vi "About Robot.vi"(8 "error in (no error)":errorcluster) -> (0 "error out":errorcluster)   [LabVIEW 2011]
panel:
  in  "stop?":bool
  in  "Tab Control":T1(tab)
  # "Autonomous Mapping Robot Platform"
  # "Robot Discription Goes Here:"
  # "Laser Range \nFinder (LIDAR)"
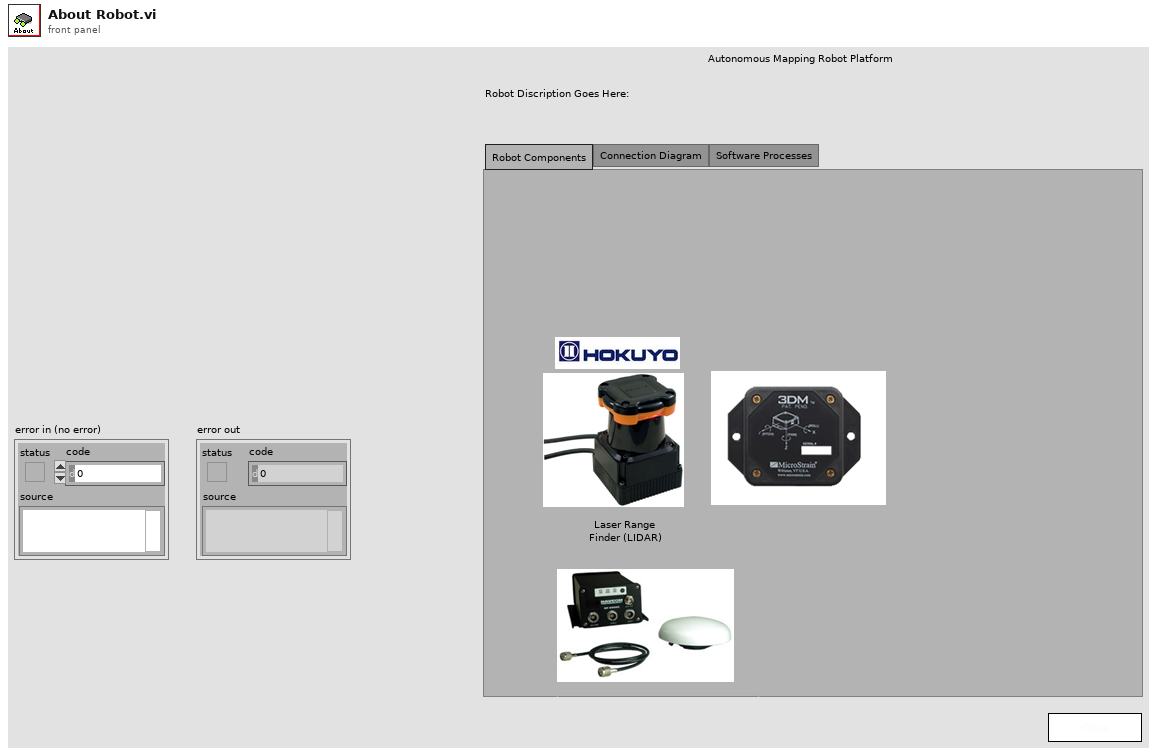
[diagram p1: front panel]
types:
  T1 = enum32{"Robot Components", "Connection Diagram", "Software Processes"}
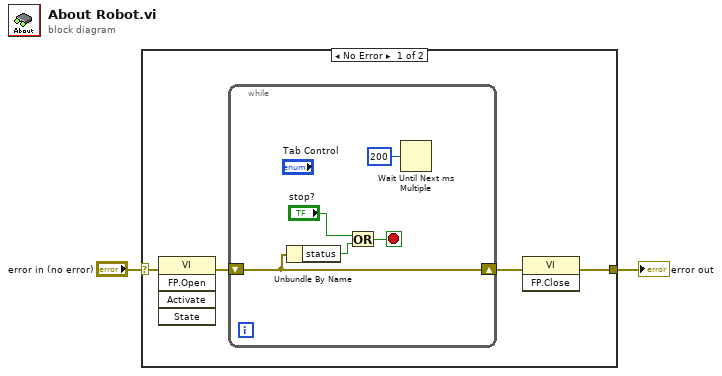
[diagram p0: block diagram]
diagram:
  n1 = case shown="No Error" "error in (no error)" {
    selector: "error in (no error)" -> [w3 w12]
    tunnel: [w4 w12] -> w2
    frame No Error {
      n2 = invoke class="VI" method="FP.Open"(error in=w3) -> (error out=w6:errorcluster)  [unwired: 4 in, 4 out]
      n3 = while {
        shift-right: [w8] -> w5
        shift-left: w6 -> [w8]
        stop <- w10 stop-if-true
        n4 = Unbundle By Name(w8) -> ("status"=w11:bool)
        n5 = Or(x="stop?", y=w11) -> (x .or. y?=w10:bool)
        n6 = Wait Until Next ms Multiple(millisecond multiple=u32 200) -> ()  [unwired: 1 out]
      }
      n7 = invoke class="VI" method="FP.Close"(error in=w5) -> (error out=w4:errorcluster)  [unwired: 2 in, 2 out]
    }
    frame Error {
    }
  }
  "error out" <- w2
